vi "nav0.vi"(9 "Drone":T4, 11 "Field":T2[][](array[typedef])) -> (2 "Move?":bool, 3 "direction":T3 items=["^", "^>", ">", "V>", "V", "<V", "<", "<^"])   [LabVIEW 2009]
uses:
  Drone data.ctl
  direction.ctl
  square.ctl
panel:
  out "ideal direction":dbl(knob) scale=0.0..8.0
  out "move matrix":bool[][](array[boolean])
  in  "Direction":T1(radio)
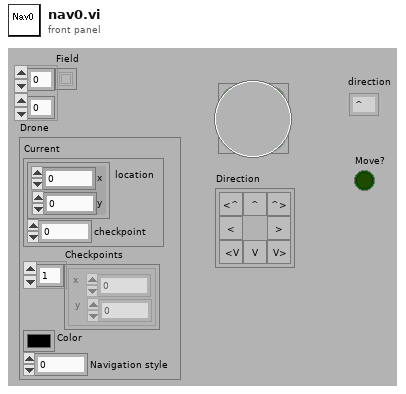
[diagram p1: front panel]
types:
  T1 = enum32{"No Selection", "dir 0", "dir 1", "dir 2", "dir 3", "dir 4", "dir 5", "dir 6", "dir 7"}
  T2 = typedef "square.ctl" = u8
  T3 = typedef "direction.ctl" = i8
  T4 = typedef "Drone data.ctl" = cluster{"Current":cluster{"location":cluster{"x":i16, "y":i16}, "checkpoint":i32}, "Checkpoints":cluster{"x":i16, "y":i16}[], "Color":u32, "Navigation style":i32}
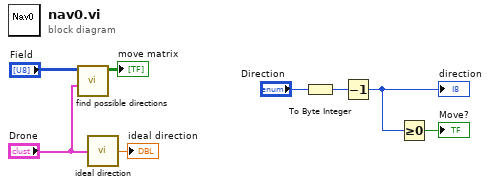
[diagram p0: block diagram]
diagram:
  n1 = call "find possible directions.vi"("Drone"="Drone", "Field"="Field") -> ("move matrix"=→"move matrix":bool[][])  [unwired: 8 in, 1 out]
  n2 = call "ideal direction.vi"("Drone"="Drone") -> ("ideal direction"=→"ideal direction":dbl)
  n3 = To Byte Integer(number="Direction") -> (8bit integer=w7:i8)
  n4 = Decrement(x=w7) -> (x-1=w6:i8)
  "direction" <- w6
  n5 = Greater Or Equal To 0?(x=w6) -> (x >= 0?=→"Move?":bool)
